vi "Manager Executable Post-Build Action.vi"(5 "Files Generated by Build":path[](array[path]), 6 "Top Level/Always Included VIs":path[](array[path]), 7 "Destination Path":path, 8 "error in (no error)":errorcluster, 9 "Target Name":string, 10 "Build Specification Name":string, 11 "Project Path":path) -> (0 "error out":errorcluster)   [LabVIEW 2021, in "CIF Manager Build Actions.lvlib"]
uses:
  CIF Manager Build Actions.lvlib
  <vilib>/regexp/Match Regular Expression.xnode
  <vilib>/CIF Foundation/CIF Utilities/File/File_CIF_U.lvlib
  <vilib>/CIF Foundation/CIF Core/CIFUtilities/CIFConfigurationFile/CIF Configuration File.lvlib
  <vilib>/CIF Foundation/CIF Core/CIFUtilities/CIFConfigurationFile/typedef/Location Type.ctl
  <vilib>/Utility/config.llb/NI_LVConfig.lvlib
  <vilib>/Utility/config.llb/Write Key (Boolean).vi
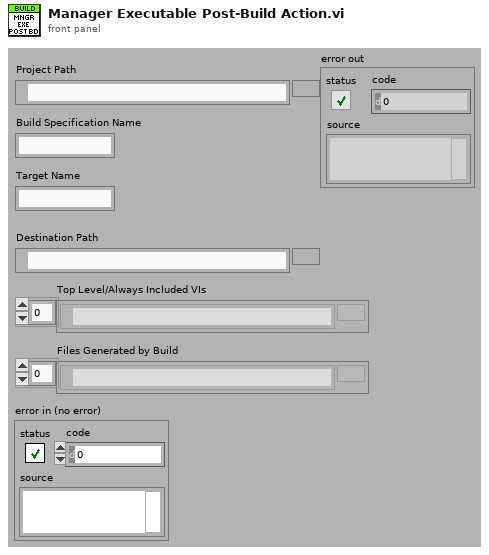
[diagram p1: front panel]
types:
  T1 = typedef "CIF Configuration File.lvlib/Location Type.ctl" = enum16{"Config File", "Manager", "Protos", "Plugins", "UI Plugins", "Logs", "Orchestrations", "Loaders"}
  T2 = typedef "NI_LVConfig.lvlib/Config Data RefNum.ctl" = refnum<k1>
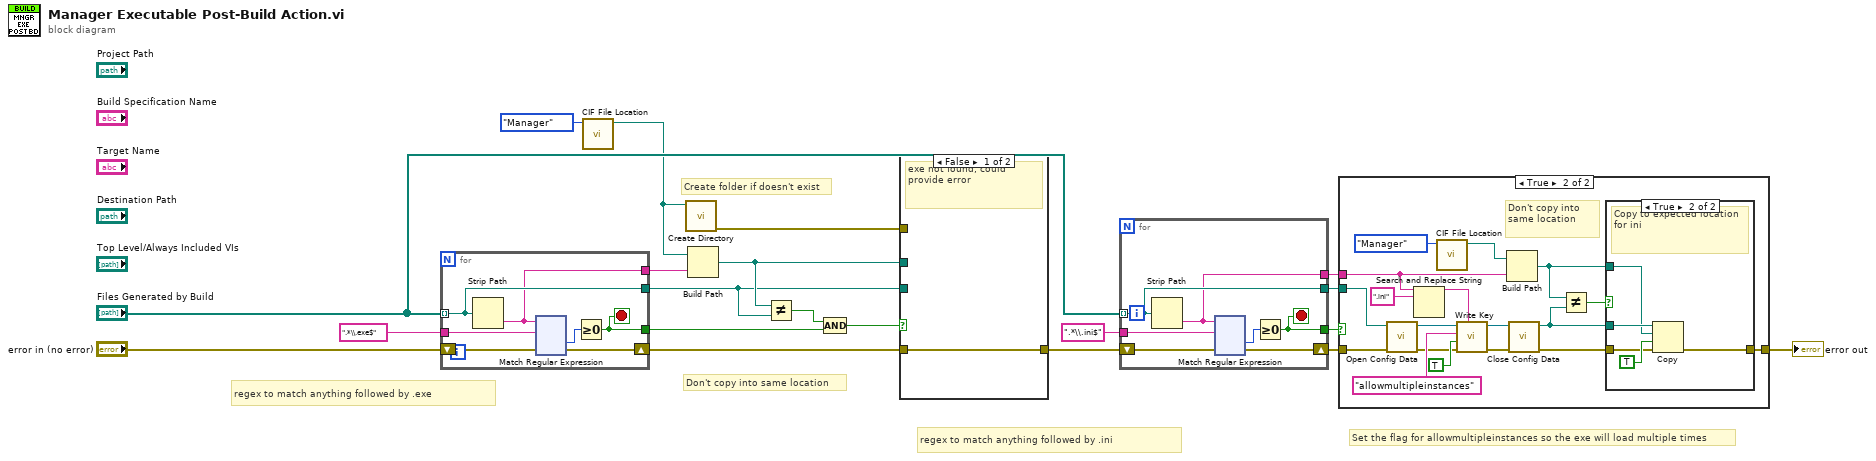
[diagram p0: block diagram]
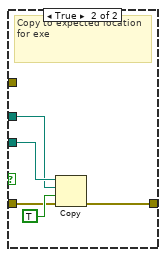
[diagram p4: hidden frame]
diagram:
  # "Set the flag for allowmultipleinstances so the exe will load multiple times"
  # "regex to match anything followed by .ini"
  # "Create folder if doesn't exist"
  # "Don't copy into same location"
  # "regex to match anything followed by .exe"
  n1 = for {
    tunnel: "Files Generated by Build" -> [w26] mode=indexing
    tunnel: ".*\\.exe$" ("pattern") -> [w27]
    tunnel: [w26] -> w15
    tunnel: [w24] -> w19
    shift-right: [w22] -> w17
    shift-left: "error in (no error)" -> [w23]
    tunnel: [w21] -> w14
    stop <- w21 stop-if-true
    n2 = Strip Path(path=w26) -> (name=w24:string)  [unwired: 1 out]
    n3 = xnode "Match Regular Expression"("input string"=w24, "regular expression"=w27, "error in"=w23) -> ("offset past match"=w25:i32, "error out"=w22:errorcluster)  [unwired: 3 in, 3 out]
    n4 = Greater Or Equal To 0?(x=w25) -> (x >= 0?=w21:bool)
  }
  n5 = call <vilib>:"CIF File Location.vi"("LocationType"=Location_Type."Manager") -> ("Location"=w4:path)  [unwired: 10 in]
  n6 = call <vilib>:"Create Directory.vi"("Path In"=w4) -> ("error out"=w11:errorcluster)  [unwired: 9 in, 1 out]
  n7 = Build Path(base path=w4, name or relative path=w19) -> (appended path=w16:path)
  n8 = Not Equal?(x=w16, y=w15) -> (x != y?=w13:bool)
  n9 = Compound Arithmetic op=AND(w13, w14) -> (w12:bool)
  n10 = case shown="False" w12 {
    tunnel: w15 -> [_ w150]
    tunnel: w16 -> [_ w149]
    tunnel: w17 -> [w145 w147]
    tunnel: [w145 w146] -> w6
    tunnel: w11 -> [_ _]
    frame False {
      # "exe not found, could provide error"
    }
    frame True {
      # "Copy to expected location for exe"
      n11 = Copy(8:w147, 9:TRUE ("overwrite (F)"), 10:w149, 11:w150) -> (0:w146:errorcluster)  [unwired: 1 in, 2 out]
    }
  }
  n12 = for {
    tunnel: "Files Generated by Build" -> [w156] mode=indexing
    tunnel: ".*\\.ini$" ("pattern") -> [w157]
    tunnel: [w156] -> w8
    tunnel: [w154] -> w3
    shift-right: [w152] -> w9
    shift-left: w6 -> [w153]
    tunnel: [w151] -> w1
    stop <- w151 stop-if-true
    n13 = Strip Path(path=w156) -> (name=w154:string)  [unwired: 1 out]
    n14 = xnode "Match Regular Expression"("input string"=w154, "regular expression"=w157, "error in"=w153) -> ("offset past match"=w155:i32, "error out"=w152:errorcluster)  [unwired: 3 in, 3 out]
    n15 = Greater Or Equal To 0?(x=w155) -> (x >= 0?=w151:bool)
  }
  n16 = case shown="True" w1 {
    tunnel: w9 -> [w275 w288]
    tunnel: w8 -> [_ w285]
    tunnel: w3 -> [_ w281]
    tunnel: [w275 w278] -> w2
    frame False {
    }
    frame True {
      # "Don't copy into same location"
      n17 = call <vilib>:"Open Config Data.vi"("error in (no error)"=w288, "configuration file path"=w285) -> ("error out"=w289:errorcluster, "refnum"=w286:T2)  [unwired: 7 in, 1 out]
      n18 = Search and Replace String(input string=w281, search string=".ini" ("substring (\"\")")) -> (result string=w291:string)  [unwired: 6 in, 3 out]
      n19 = call <vilib>:"CIF File Location.vi"("LocationType"=Location_Type."Manager") -> ("Location"=w276:path)  [unwired: 10 in]
      n20 = call-poly <vilib>:"Write Key.vi"("section"=w291, "error in (no error)"=w289, "value"=TRUE, "key"="allowmultipleinstances", "refnum"=w286) -> ("error out"=w284:errorcluster, "refnum out"=w287:T2)  [unwired: 4 in, 1 out]
      n21 = Build Path(base path=w276, name or relative path=w281) -> (appended path=w283:path)
      n22 = call <vilib>:"Close Config Data.vi"("error in (no error)"=w284, "refnum"=w287) -> ("error out"=w282:errorcluster, "file path"=w280:path)  [unwired: 8 in]
      n23 = Not Equal?(x=w283, y=w280) -> (x != y?=w279:bool)
      n24 = case shown="True" w279 {
        tunnel: w280 -> [_ w299]
        tunnel: w283 -> [_ w298]
        tunnel: w282 -> [w294 w296]
        tunnel: [w294 w295] -> w278
        frame False {
          # "ini not found, could provide error"
        }
        frame True {
          # "Copy to expected location for ini"
          n25 = Copy(8:w296, 9:TRUE ("overwrite (F)"), 10:w298, 11:w299) -> (0:w295:errorcluster)  [unwired: 1 in, 2 out]
        }
      }
    }
  }
  "error out" <- w2
